vi "DK240 GratingInfo.vi"(6 "error in":errorcluster, 8 "Port":refnum<visa-resource-name>="SPECTRO") -> (0 "error out":errorcluster, 1 "Mirr":u16 caption="Mirroitement(nm)" step=1, 2 "Status":u8, 3 "Rés act":u8 caption="Réseau Act", 4 "l/mm":u16 caption="Ligne/mm" step=1, 5 "Nb Rés":u8 caption="Nb Réseaux" max=3 step=1)   [LabVIEW 2019]
doc: "Ce VI retourne les informations sur le réseaux actuel, soit son numéro, son pas, sa longueur d'onde de mirroitement ainsi que le nombre totale de réseaux installé."
uses:
  <vilib>/Utility/error.llb/DialogType.ctl
panel:
  out "Cancel":u8
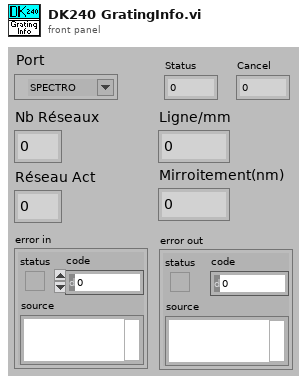
[diagram p1: front panel]
types:
  T1 = typedef "DialogType.ctl" = u16
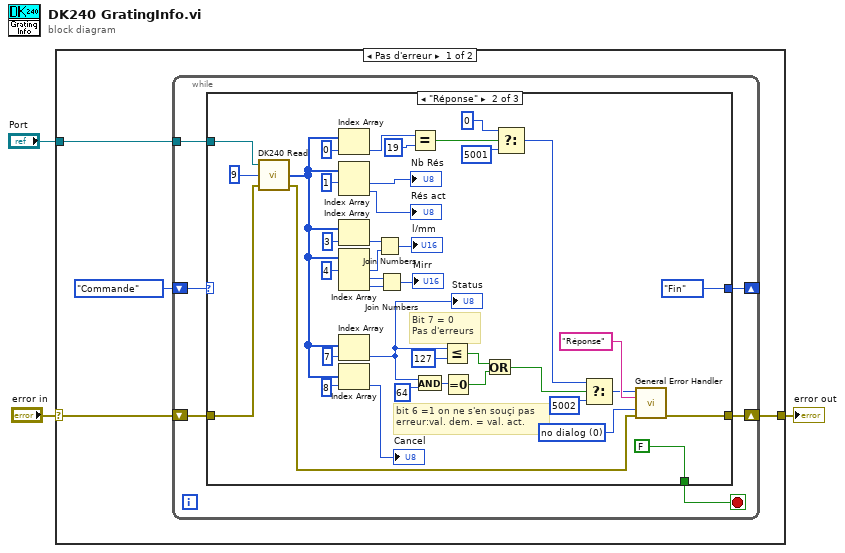
[diagram p0: block diagram]
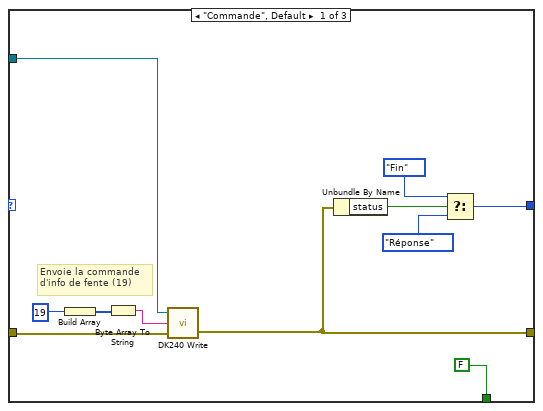
[diagram p2: hidden frame]
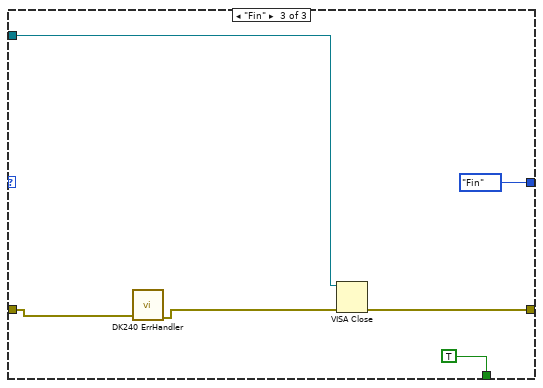
[diagram p3: hidden frame]
diagram:
  n1 = case shown="Pas d'erreur" "error in" {
    selector: "error in" -> [w4 w71]
    tunnel: "Port" -> [w7 _]
    tunnel: [w6 w71] -> w2
    frame No Error {
      n2 = while {
        tunnel: w7 -> [w12]
        shift-right: [w10] -> w6
        shift-left: w4 -> [w11]
        shift-right: [w8] -> _
        shift-left: enum16{"Commande", "Réponse", "Fin"}."Commande" -> [w9]
        stop <- w13 stop-if-true
        n3 = case shown="\"Réponse\"" w9 {
          tunnel: [FALSE FALSE TRUE] -> w13
          tunnel: w12 -> [w20 w58 w68]
          tunnel: w11 -> [w19 w57 w66]
          tunnel: [w16 w44 w67] -> w10
          tunnel: [w14 enum16{"Commande", "Réponse", "Fin"}."Fin" enum16{"Commande", "Réponse", "Fin"}."Fin"] -> w8
          frame "Commande", Default {
            # "Envoie la commande\nd'info de fente (19)"
            n4 = Build Array(u8 19) -> (w24:u8[])
            n5 = Byte Array To String(unsigned byte array=w24) -> (string=w21:string)
            n6 = call <userlib>:"DK240 Write.vi"("error in"=w19, "String to write"=w21, "Port"=w20) -> ("error out"=w16:errorcluster)  [unwired: 1 in]
            n7 = Unbundle By Name(w16) -> ("status"=w15:bool)
            n8 = Select(t=enum16{"Commande", "Réponse", "Fin"}."Fin", s=w15, f=enum16{"Commande", "Réponse", "Fin"}."Réponse") -> (s? t:f=w14:enum16{"Commande", "Réponse", "Fin"})
          }
          frame "Réponse" {
            w50 = T1 0 items=["no dialog", "OK message", "continue or stop message", "OK message + warnings", "continue/stop + warnings"] ("type of dialog (OK msg:1)")
            # "bit 6 =1 on ne s'en souçi pas \nerreur:val. dem. = val. act."
            # "Bit 7 = 0\nPas d'erreurs"
            n9 = call <userlib>:"DK240 Read.vi"("error in"=w57, "Byte count"=u32 9, "Port"=w58) -> ("error out"=w45:errorcluster, "Received Bytes"=w41:u8[])  [unwired: 1 in]
            n10 = Index Array(array=w41, index=0) -> (element=w37:u8)
            n11 = Index Array(array=w41, index #1=1) -> (element #1=→"Nb Rés":u8, element #2=→"Rés act":u8)  [unwired: 1 in]
            n12 = Index Array(array=w41, index=3) -> (element=w31:u8)
            n13 = Index Array(array=w41, index #1=4) -> (element #1=w30:u8, element #2=w27:u8, element #3=w28:u8)  [unwired: 2 in]
            n14 = Index Array(array=w41, index=7) -> (element=w33:u8)
            "Status" <- w33
            n15 = Index Array(array=w41, index=8) -> (element=→"Cancel":u8)
            n16 = Join Numbers(hi=w31, lo=w30) -> ((hi.lo)=→"l/mm":u16)
            n17 = Join Numbers(hi=w27, lo=w28) -> ((hi.lo)=→"Mirr":u16)
            n18 = Equal?(x=w37, y=u8 19) -> (x = y?=w35:bool)
            n19 = And(x=w33, y=u8 64) -> (x .and. y?=w52:u8)
            n20 = Less Or Equal?(x=w33, y=u8 127) -> (x <= y?=w53:bool)
            n21 = Equal To 0?(x=w52) -> (x = 0?=w54:bool)
            n22 = Or(x=w53, y=w54) -> (x .or. y?=w55:bool)
            n23 = Select(t=0, s=w35, f=5001 ("t")) -> (s? t:f=w34:i32)
            n24 = Select(t=w34, s=w55, f=5002 ("t")) -> (s? t:f=w47:i32)
            n25 = call <vilib>:"General Error Handler.vi"("[error code] (0)"=w47, "[error source] (\" \")"="Réponse" ("[error source] (\" \")"), "type of dialog (OK msg:1)"=w50, "error in (no error)"=w45) -> ("error out"=w44:errorcluster)  [unwired: 7 in, 4 out]
          }
          frame "Fin" {
            n26 = call <userlib>:"DK240 ErrHandler.vi"("error in"=w66) -> ("error out"=w65:errorcluster)  [unwired: 7 in]
            n27 = VISA Close(VISA resource name=w68, error in (no error)=w65) -> (error out=w67:errorcluster)
          }
        }
      }
    }
    frame Error {
    }
  }
  "error out" <- w2
